vi "Add to IG time array.vi"(1 "Record Max Size":i32, 2 "timestamp in seconds from 1904":dbl, 3 "IG Value":dbl, 4 "IGvsTime Array In":dbl[][](array[numeric])) -> (0 "IGvsTime Array Out":dbl[][](array[numeric]))   [LabVIEW 2016]
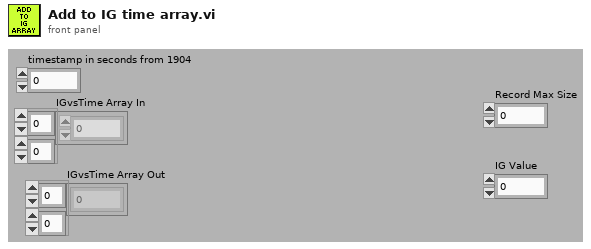
[diagram p1: front panel]
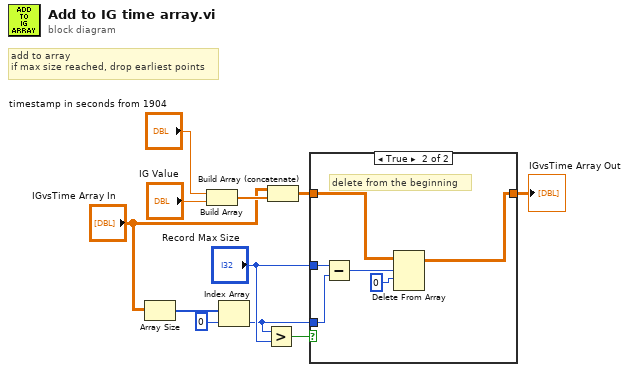
[diagram p0: block diagram]
diagram:
  # "add to array\nif max size reached, drop earliest points"
  n1 = Array Size(array="IGvsTime Array In") -> (size(s)=w3:i32[])
  n2 = Build Array("timestamp in seconds from 1904", "IG Value") -> (w8:dbl[])
  n3 = Index Array(array=w3, index=0) -> (element=w1:i32)
  n4 = Greater?(x=w1, y="Record Max Size") -> (0:w11:bool)
  n5 = Build Array (concatenate)("IGvsTime Array In", w8) -> (w10:dbl[][])
  n6 = case shown="True" w11 {
    tunnel: w10 -> [w12 w18]
    tunnel: "Record Max Size" -> [_ w16]
    tunnel: w1 -> [_ w15]
    tunnel: [w12 w13] -> w6
    frame False {
    }
    frame True {
      # "delete from the beginning"
      n7 = Subtract(x=w16, y=w15) -> (x-y=w14:i32)
      n8 = Delete From Array(array=w18, length=w14, index (row)=0 ("index")) -> (array with subset deleted=w13:dbl[][])  [unwired: 1 in, 1 out]
    }
  }
  "IGvsTime Array Out" <- w6
